vi "serverID.vi"() -> ()   [LabVIEW 2013, in "udplib.lvlib"]
uses:
  udplib.lvlib
panel:
  out "ServerIDout":u8
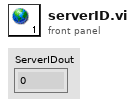
[diagram p1: front panel]
diagram:
